vi "SM_S700_Serial_String_to_timestamp.vi"(8 "error in (no error)":errorcluster, 10 "initial scan location":u32, 11 "read buffer":string) -> (0 "error out":errorcluster, 2 "Time Stamp":timestamp, 3 "String":string)   [LabVIEW 2011]
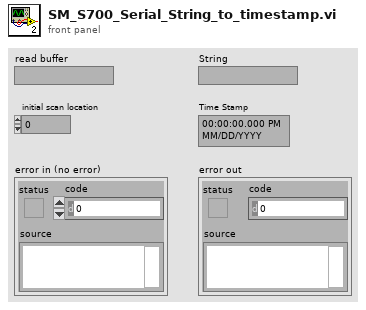
[diagram p1: front panel]
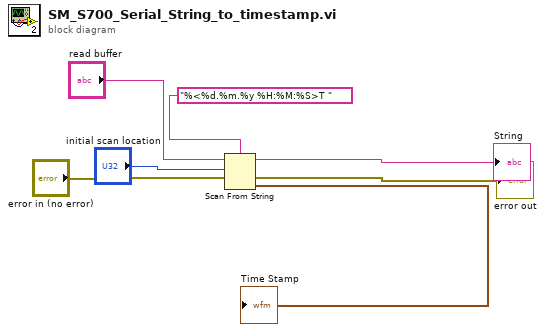
[diagram p0: block diagram]
diagram:
  n1 = Scan From String(format string="%<%d.%m.%y %H:%M:%S>T ", input string="read buffer", initial scan location="initial scan location", error in="error in (no error)") -> (remaining string=→"String":string, error out=→"error out":errorcluster, output 1=→"Time Stamp":timestamp)  [unwired: 1 in, 1 out]
